vi "io废.vi"() -> ()   [LabVIEW 2020]
uses:
  <vilib>/Platform/TimedLoop/XDataNode/timing_clust.ctl
  <vilib>/Platform/TimedLoop/XDataNode/nitl_modes.ctl
  <vilib>/Platform/TimedLoop/XDataNode/wakeup.ctl
  <vilib>/FPGAPlugInAG/cRIO-9047/niLvFpga_Open_cRIO-9047.vi
  <vilib>/rvi/interface/common/dynamic/niFpgaDynamicAddResources.vi
  <vilib>/FPGAPlugInAG/Dynamic/niLvFpga_Download_Dynamic.vi
  <vilib>/FPGAPlugInAG/Dynamic/niLvFpga_Reset_Dynamic.vi
  <vilib>/FPGAPlugInAG/Dynamic/niLvFpga_Run_Dynamic.vi
  <vilib>/Utility/error.llb/Error Cluster From Error Code.vi
  <vilib>/rvi/errors/niLvFpgaAdjustHostInterfaceError.vi
  <vilib>/FPGAPlugInAG/Dynamic/niLvFpga_Close_Dynamic.vi
  <vilib>/rvi/interface/nirviOpenFPGA/nirviOpenFPGA.xnode
  testFPGA/FPGA_main.vi
  <vilib>/rvi/interface/nirviMethod/nirviMethod.xnode
  <vilib>/Platform/TimedLoop/XDataNode/XDataNode.xnode
  <vilib>/rvi/interface/nirviReadWriteControl/nirviReadWriteControl.xnode
  <vilib>/rvi/interface/nirviCloseFPGA/nirviCloseFPGA.xnode
  FPGA_Motor_IO.vi
  <vilib>/Platform/TimedLoop/XDataNode/XDNodeRunTimeDep.lvlib
  NiFpgaLv.dll
  <vilib>/rvi/interface/Simulation/niFpgaSimulationCallBeginRW.vi
panel:
  in  "frequency (periods/tick) 2":fxp<+,32,0>=2.4999957531690598e-05
  in  "duty cycle (periods) 2":fxp<+,32,0>=0.10000000009313226
  in  "Direction 2":bool
  in  "POWER OFF 2":bool=TRUE
  in  "Enable 2":bool
  out "SensorV":dbl(graph)
  out "cmArrayBody1":dbl[](array[numeric])
  out "XYZ":T1(graph)
  out "Theta":dbl(graph)
  out "Length":dbl(graph)
  out "Phi":dbl(graph)
  out "Pressure":dbl(graph)
  out "Q":dbl(graph)
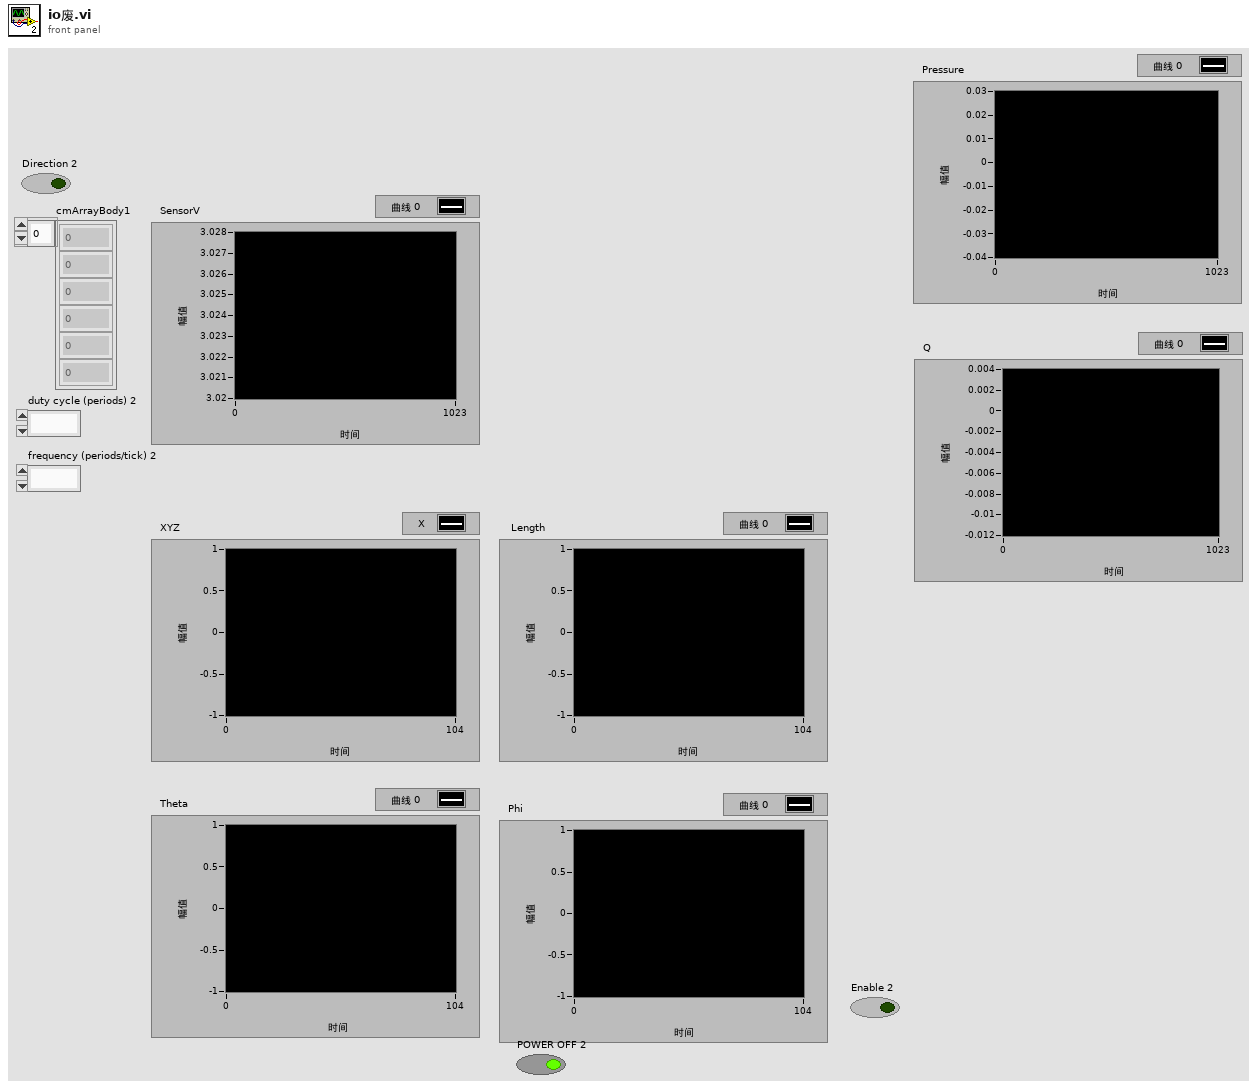
[diagram p1: front panel]
types:
  T1 = cluster{"Numeric":dbl, "Numeric":dbl, "Numeric":dbl}
  T2 = typedef "XDNodeRunTimeDep.lvlib/timing_clust.ctl" = cluster{"Expected End [f-1]":u64, "Actual End [f-1]":u64, "Finished Late? [f-1]":bool, "Expected End [i-1]":u64, "Actual End [i-1]":u64, "Finished Late? [i-1]":bool, "Expected Start [i]":u64, "Actual Start [i]":u64, "Expected Start [f]":u64, "Actual Start [f]":u64, "Source Name":string, "Structure Name":string, "Period":i64, "Deadline":i64, "Offset":i64, "Start":i64, "Priority":i32, "Timeout":i32, "Mode":T3, "Wakeup Reason":T4, "Error":errorcluster, "Source Type":string, "Secondary Source Type":string, "Global End Time":u64, "Global Start Time":u64, "Frame Duration":u64, "Iteration Duration":u64, "Assigned CPU":i32, "I/O Scan Engine Mode":u32}
  T3 = typedef "XDNodeRunTimeDep.lvlib/nitl_modes.ctl" = enum32{"No Change", "Process missed periods, maintain original phase", "Discard missed periods, maintain original phase", "Process missed periods, ignore original phase", "Discard missed periods, ignore original phase"}
  T4 = typedef "XDNodeRunTimeDep.lvlib/wakeup.ctl" = enum32{"Normal", "Aborted", "Asynchronous wakeup", "Timing source error", "Timed loop error", "Timeout"}
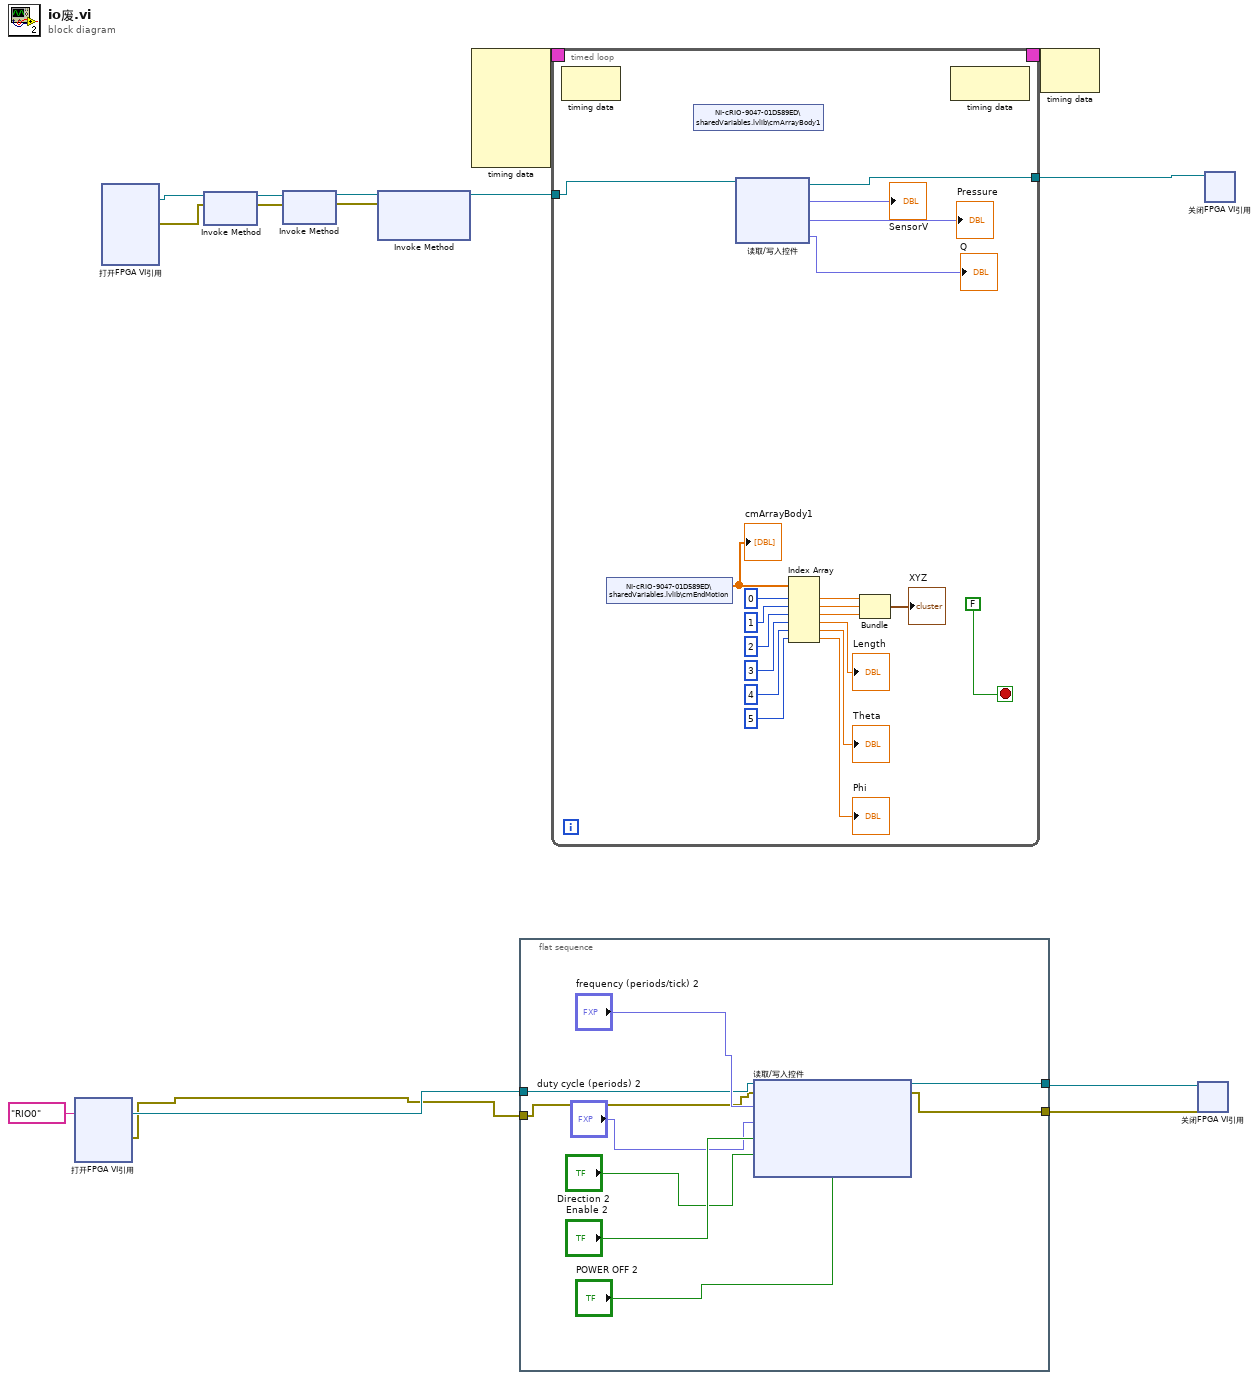
[diagram p0: block diagram]
diagram:
  n1 = xnode "打开FPGA VI引用"("资源名称"=tag "RIO0") -> ("FPGA VI引用输出"=w2:refnum<k20>, "错误输出"=w1:errorcluster)  [unwired: 1 in]
  n2 = xnode "打开FPGA VI引用"() -> ("FPGA VI引用输出"=w12:refnum<k20>, "错误输出"=w13:errorcluster)  [unwired: 2 in]
  n3 = xnode "Invoke Method"("FPGA VI引用输入"=w12, "错误输入"=w13) -> ("FPGA VI引用输出"=w11:refnum<k20>, "错误输出"=w10:errorcluster)
  n4 = xnode "Invoke Method"("FPGA VI引用输入"=w11, "错误输入"=w10) -> ("FPGA VI引用输出"=w8:refnum<k20>, "错误输出"=w9:errorcluster)
  n5 = xnode "Invoke Method"("FPGA VI引用输入"=w8, "错误输入"=w9) -> ("FPGA VI引用输出"=w7:refnum<k20>)  [unwired: 1 in, 1 out]
  n6 = node-c288() -> (w15:T2)  [unwired: 6 in]
  n7 = flat-sequence {
    tunnel: w2 -> [w18]
    tunnel: [w19] -> w5
    tunnel: w1 -> [w17]
    tunnel: [w16] -> w3
    frame #0 {
      n8 = xnode "读取/写入控件"("FPGA VI引用输入"=w18, "错误输入"=w17, "frequency (periods/tick)"="frequency (periods/tick) 2", "duty cycle (periods)"="duty cycle (periods) 2", "Enable"="Enable 2", "Direction"="Direction 2", "POWER OFF"="POWER OFF 2") -> ("FPGA VI引用输出"=w19:refnum<k20>, "错误输出"=w16:errorcluster)
    }
  }
  n9 = timed-loop {
    timing: w15 -> [_]
    timing-out: [_] -> w14
    tunnel: w7 -> [w44]
    tunnel: [w43] -> w6
    stop <- FALSE stop-if-true
    n10 = node-c288() -> ()  [unwired: 1 in, 1 out]
    n11 = shared-variable "NI-cRIO-9047-01D589ED\\sharedVariables.lvlib\\cmEndMotion"() -> (w41:dbl[])  [unwired: 1 in, 1 out]
    "cmArrayBody1" <- w41
    n12 = shared-variable "NI-cRIO-9047-01D589ED\\sharedVariables.lvlib\\cmArrayBody1"() -> ()  [unwired: 1 in, 2 out]
    n13 = xnode "读取/写入控件"("FPGA VI引用输入"=w44) -> ("FPGA VI引用输出"=w43:refnum<k20>, "Encoder1"=→"SensorV":fxp<+/-,24,5>, "Pressure"=→"Pressure":fxp<+/-,24,5>, "Q"=→"Q":fxp<+/-,24,5>)  [unwired: 1 in, 1 out]
    n14 = Index Array(array=w41, index #1=0, index #2=1, index #3=2, index #4=3, index #5=4, index #6=5) -> (element #1=w34:dbl, element #2=w33:dbl, element #3=w32:dbl, element #4=→"Length":dbl, element #5=→"Theta":dbl, element #6=→"Phi":dbl)
    n15 = Bundle("Numeric"=w34, "Numeric"=w33, "Numeric"=w32) -> (→"XYZ":T1)  [unwired: 1 in]
    n16 = node-c288() -> ()  [unwired: 1 in, 1 out]
  }
  n17 = node-c288(w14) -> ()  [unwired: 1 out]
  n18 = xnode "关闭FPGA VI引用"("FPGA VI引用输入"=w5, "错误输入"=w3) -> ()  [unwired: 1 out]
  n19 = xnode "关闭FPGA VI引用"("FPGA VI引用输入"=w6) -> ()  [unwired: 1 in, 1 out]
